vi "flux.vi"(1 "dt":dbl, 2 "Membrane Area":dbl=1.0, 3 "dV":dbl) -> (0 "Avg. Flux":dbl)   [LabVIEW 2015]
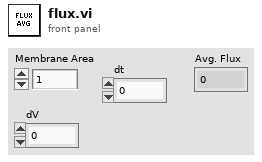
[diagram p1: front panel]
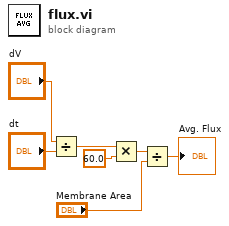
[diagram p0: block diagram]
diagram:
  n1 = Divide(x="dV", y="dt") -> (x/y=w3:dbl)
  n2 = Multiply(x=w3, y=60.0) -> (x*y=w5:dbl)
  n3 = Divide(x=w5, y="Membrane Area") -> (x/y=→"Avg. Flux":dbl)
